vi "get checkpoint step size.vi"(8 "error in (no error)":errorcluster, 11 "Autofocus in":refnum<class "Autofocus.lvclass">) -> (0 "error out":errorcluster, 2 "checkpoint stepsize":dbl[unit], 3 "Autofocus out":refnum<class "Autofocus.lvclass">)   [LabVIEW 2012, in "Autofocus.lvclass"]
uses:
  Autofocus.lvclass
  Autofocus.lvclass/Autofocus.ctl
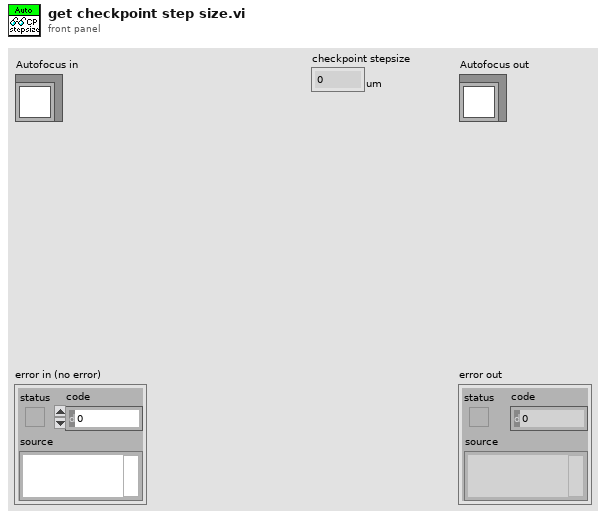
[diagram p1: front panel]
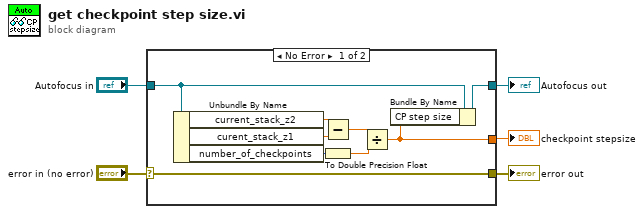
[diagram p0: block diagram]
diagram:
  n1 = case shown="No Error" "error in (no error)" {
    selector: "error in (no error)" -> [w14 w16]
    tunnel: [w14 w16] -> w4
    tunnel: [w7 w15] -> w2
    tunnel: "Autofocus in" -> [w8 w15]
    tunnel: [w6 _] -> w1
    frame No Error {
      n2 = Unbundle By Name(w8) -> ("current_stack_z2"=w13:dbl[unit], "curent_stack_z1"=w12:dbl[unit], "number_of_checkpoints"=w10:u16)
      n3 = Subtract(x=w13, y=w12) -> (x-y=w11:dbl[unit])
      n4 = To Double Precision Float(number=w10) -> (double precision float=w9:dbl)
      n5 = Divide(x=w11, y=w9) -> (x/y=w6:dbl[unit])
      n6 = Bundle By Name(cluster=w8, "CP step size"=w6) -> (w7:refnum<class "Autofocus.lvclass">)
    }
    frame Error {
    }
  }
  "error out" <- w4
  "Autofocus out" <- w2
  "checkpoint stepsize" <- w1
